vi "SMTP Email Header Word Must Be Escaped.vi"(1 "word":string) -> (0 "escape word":bool)   [LabVIEW 2011, in "NewNI_SMTPEmail.lvlib"]
uses:
  NewNI_SMTPEmail.lvlib
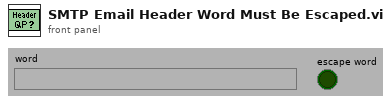
[diagram p1: front panel]
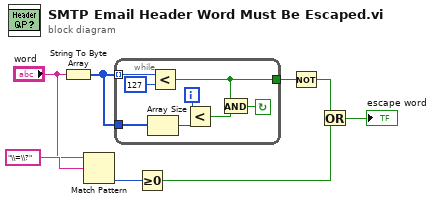
[diagram p0: block diagram]
diagram:
  n1 = String To Byte Array(string="word") -> (unsigned byte array=w7:u8[])
  n2 = Match Pattern(string="word", regular expression="\\=\\?") -> (offset past match=w4:i32)  [unwired: 4 out]
  n3 = while {
    tunnel: [w9] -> w8
    tunnel: w7 -> [w12]
    tunnel: w7 -> [w11] mode=indexing
    i -> [w16]
    stop <- w13 continue-if-true
    n4 = Array Size(array=w12) -> (size(s)=w15:i32)
    n5 = Less?(x=w11, y=u8 127) -> (x < y?=w9:bool)
    n6 = Less?(x=w16, y=w15) -> (x < y?=w14:bool)
    n7 = And(x=w9, y=w14) -> (x .and. y?=w13:bool)
  }
  n8 = Greater Or Equal To 0?(x=w4) -> (x >= 0?=w2:bool)
  n9 = Not(x=w8) -> (.not. x?=w3:bool)
  n10 = Or(x=w3, y=w2) -> (x .or. y?=→"escape word":bool)
